vi "student_error_detect_Ahmed.vi"(4 "error in (no error)":errorcluster, 6 "key bit sequence":u8[](array[numeric]), 7 "input bit sequence":u8[](array[numeric])) -> (0 "error out":errorcluster, 3 "bit-error rate":dbl)   [LabVIEW 2018]
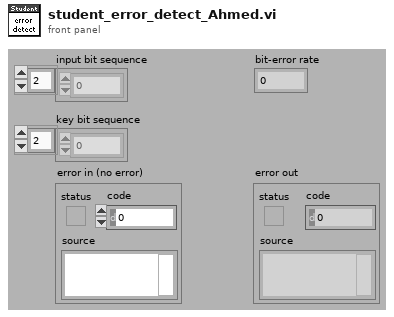
[diagram p1: front panel]
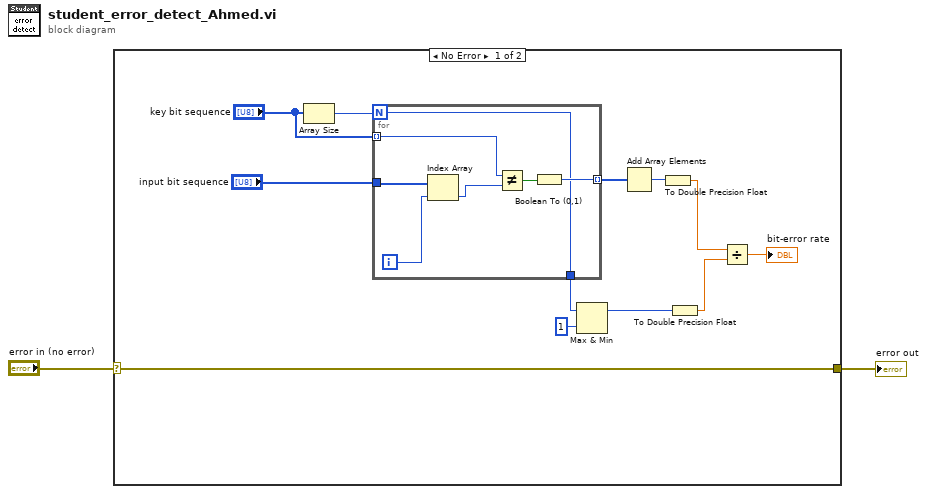
[diagram p0: block diagram]
diagram:
  n1 = case shown="No Error" "error in (no error)" {
    selector: "error in (no error)" -> [w3 w22]
    tunnel: [w3 w22] -> w2
    frame No Error {
      n2 = Array Size(array="key bit sequence") -> (size(s)=w14:i32)
      n3 = for {
        N: w14 -> [w17]
        tunnel: "key bit sequence" -> [w20] mode=indexing
        tunnel: "input bit sequence" -> [w15]
        tunnel: [w18] -> w10 mode=indexing
        tunnel: [w17] -> w8
        i -> [w16]
        n4 = Index Array(array=w15, index=w16) -> (element=w21:u8)
        n5 = Not Equal?(x=w20, y=w21) -> (x != y?=w19:bool)
        n6 = Boolean To (0,1)(Boolean=w19) -> (0, 1=w18:i16)
      }
      n7 = Max & Min(x=w8, y=1) -> (max(x,y)=w7:i32)  [unwired: 1 out]
      n8 = Add Array Elements(numeric array=w10) -> (sum=w9:i16)
      n9 = To Double Precision Float(number=w9) -> (double precision float=w6:dbl)
      n10 = To Double Precision Float(number=w7) -> (double precision float=w5:dbl)
      n11 = Divide(x=w6, y=w5) -> (x/y=→"bit-error rate":dbl)
    }
    frame Error {
    }
  }
  "error out" <- w2
